vi "mxwScript_API_XMLTemplateName_AddDropInto.vi"(8 "error in (no error)":errorcluster, 10 "diagramID":string, 11 "absolutePath":string) -> (0 "error out":errorcluster, 3 "encoded absolutePath":string)   [LabVIEW 2017]
doc: "Add diagram to drop this template into to the template name."
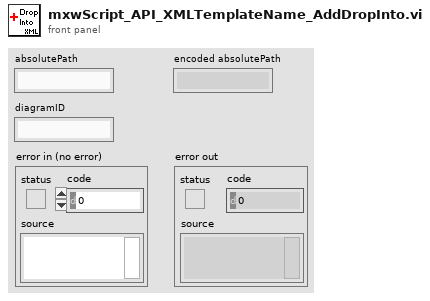
[diagram p1: front panel]
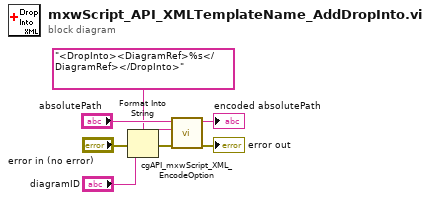
[diagram p0: block diagram]
diagram:
  n1 = Format Into String(format string="<DropInto><DiagramRef>%s</DiagramRef></DropInto>" ("control name"), error in="error in (no error)", "diagramID") -> (resulting string=w2:string, error out=w4:errorcluster)  [unwired: 1 in]
  n2 = call "cgAPI_mxwScript_XML_EncodeOption.vi"("error in (no error)"=w4, "otherXML"=w2, "normalTextString"="absolutePath") -> ("error out"=→"error out":errorcluster, "encodedString"=→"encoded absolutePath":string)  [unwired: 7 out]
